vi "MongoDB.Connection.Close.vi"(8 "error in (no error)":errorcluster, 11 "MongoDB in":refnum<class "MongoDB.Client.lvclass">) -> (0 "error out":errorcluster)   [LabVIEW 2014, in "MongoDB.Client.lvclass"]
uses:
  MongoDB.Client.lvclass
  MongoDB.Client.lvclass/MongoDB.Client.ctl
  C:/Users/Richard/Documents/GitHub/mongo-labview-driver/CSharp/bin/MongoDB.Driver.Legacy.dll
  CSharp/bin/MongoDB.Driver.Legacy.dll
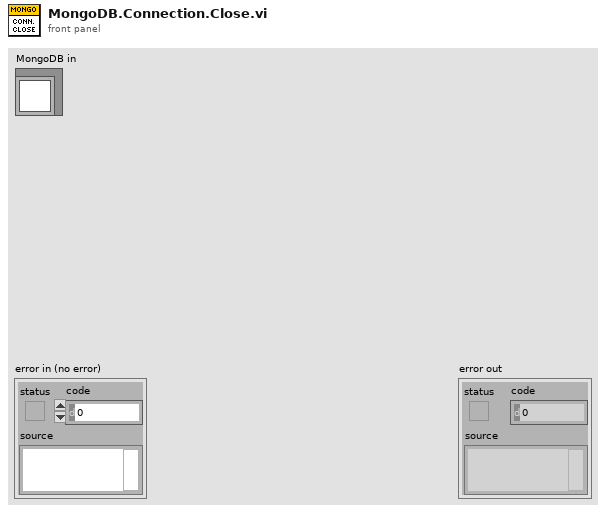
[diagram p1: front panel]
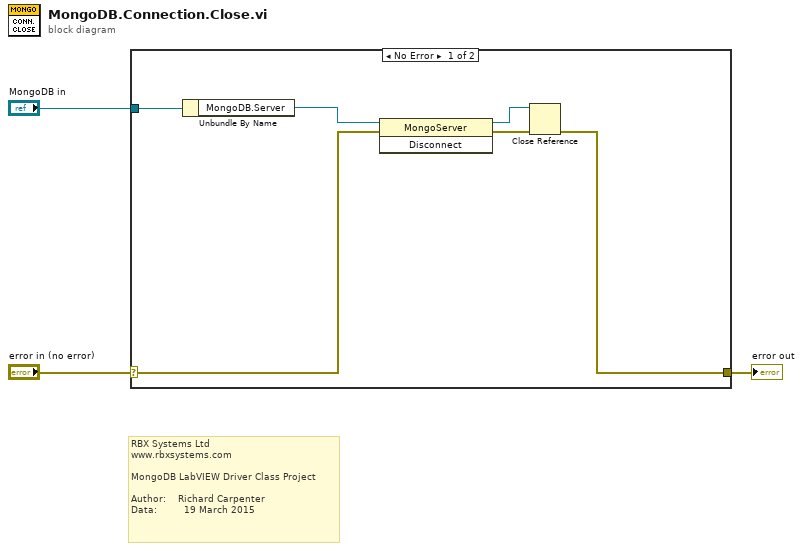
[diagram p0: block diagram]
diagram:
  # "RBX Systems Ltd\nwww.rbxsystems.com\n\nMongoDB LabVIEW Driver Class Project\n\nAuthor:    Richard Carpenter\nData:         19 March 2015"
  n1 = case shown="No Error" "error in (no error)" {
    selector: "error in (no error)" -> [w6 w10]
    tunnel: [w4 w10] -> w2
    tunnel: "MongoDB in" -> [w5 _]
    frame No Error {
      n2 = Unbundle By Name(w5) -> ("MongoDB.Server"=w9:refnum<k24>)
      n3 = invoke class="MongoServer" method="Disconnect"(reference=w9, error in=w6) -> (reference out=w8:refnum<k24>, error out=w7:errorcluster)  [unwired: 1 in, 1 out]
      n4 = Close Reference(reference=w8, error in (no error)=w7) -> (error out=w4:errorcluster)
    }
    frame Error {
    }
  }
  "error out" <- w2
